vi "Interleaver.vi"(0 "appended path":path, 5 "rm_data":dbl[][](array[numeric]), 7 "EN_INTERWEAVER":dbl, 9 "rm_len":dbl[](array[numeric]), 11 "Qm":dbl, 12 "error in (no error)":errorcluster caption="错误输入（无错误）", 13 "C":dbl) -> (1 "error out":errorcluster caption="错误输出", 14 "iw_data":dbl[][](array[numeric]))   [LabVIEW 2015]
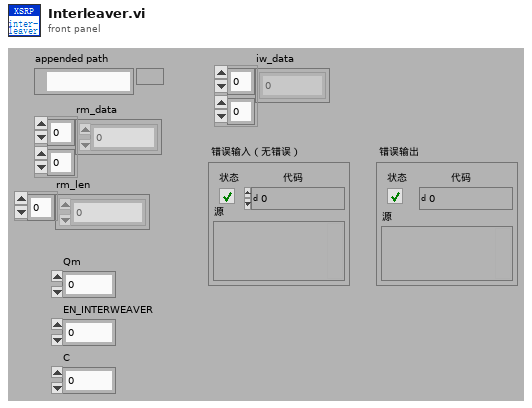
[diagram p1: front panel]
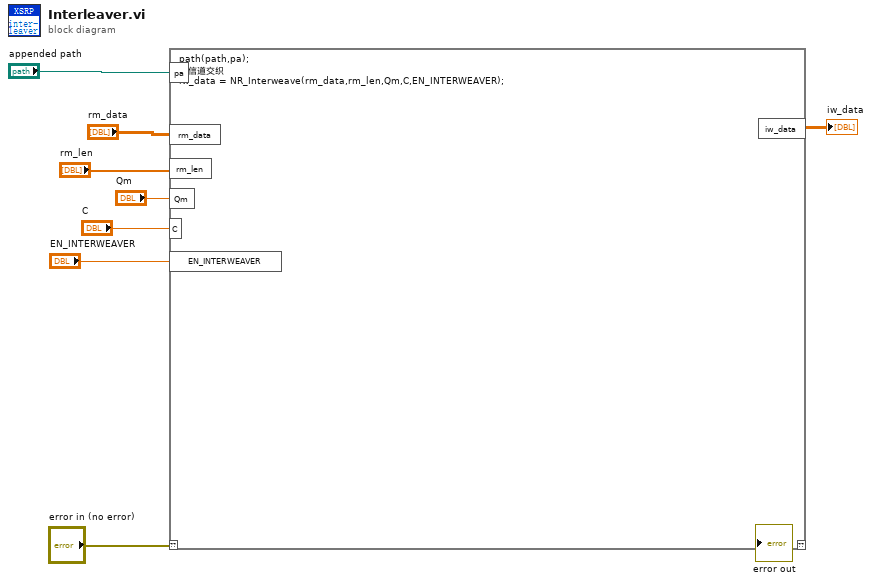
[diagram p0: block diagram]
diagram:
  n1 = script code="path(path,pa);\n%信道交织\niw_data = NR_Interweave(rm_data,rm_len,Qm,C,EN_INTERWEAVER);"("??"="error in (no error)", "pa"="appended path", "rm_data"="rm_data", "rm_len"="rm_len", "Qm"="Qm", "C"="C", "EN_INTERWEAVER"="EN_INTERWEAVER") -> ("??"=→"error out":errorcluster, "iw_data"=→"iw_data":dbl[][])
